vi "FormatWaveforms.vi"(0 "WaveformArray":sgl[](array[numeric]), 5 "logFileRef":refnum<k34>, 7 "log":bool, 9 "StreamHeader":T1, 11 "error in (no error)":errorcluster) -> (4 "Waveforms":sgl[][](array[numeric]), 6 "UpdateWaveforms":bool, 15 "error out":errorcluster)   [LabVIEW 2017]
uses:
  Controller/Support/StreamHeader.ctl
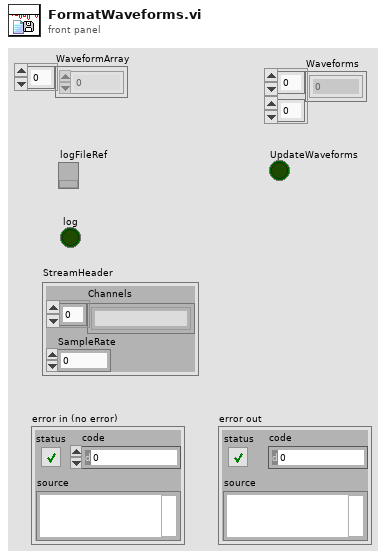
[diagram p1: front panel]
types:
  T1 = typedef "StreamHeader.ctl" = cluster{"Channels":string[], "SampleRate":i32}
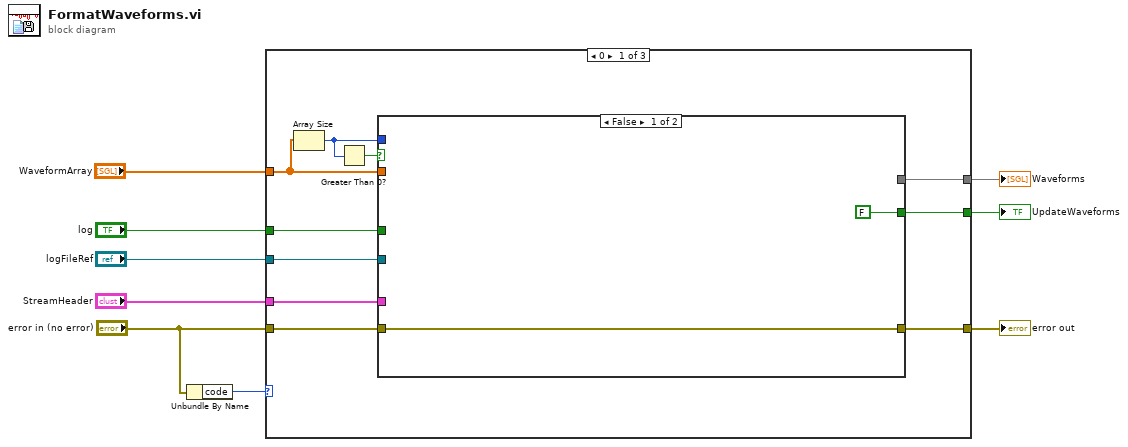
[diagram p0: block diagram]
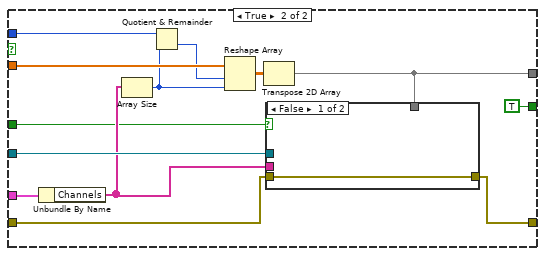
[diagram p2: hidden frame]
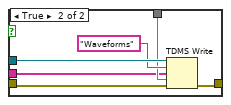
[diagram p3: hidden frame]
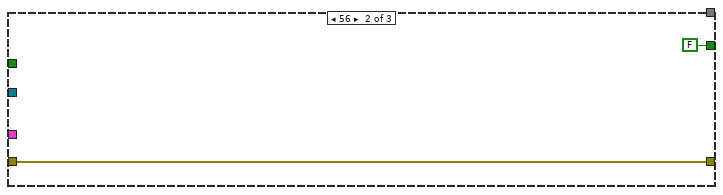
[diagram p4: hidden frame]
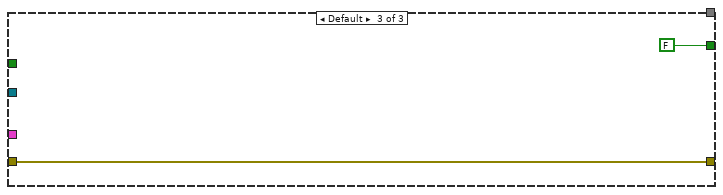
[diagram p5: hidden frame]
diagram:
  n1 = Unbundle By Name("error in (no error)") -> ("code"=w5:i32)
  n2 = case shown="0" w5 {
    tunnel: [w14 w43 w45] -> w3
    tunnel: "WaveformArray" -> [w19 _ _]
    tunnel: "StreamHeader" -> [w13 _ _]
    tunnel: "error in (no error)" -> [w15 w43 w45]
    tunnel: "logFileRef" -> [w16 _ _]
    tunnel: "log" -> [w12 _ _]
    tunnel: [w11 _ _] -> w1
    tunnel: [w10 FALSE FALSE] -> w2
    frame 0 {
      n3 = Array Size(array=w19) -> (size(s)=w18:i32)
      n4 = Greater Than 0?(x=w18) -> (x > 0?=w17:bool)
      n5 = case shown="False" w17 {
        tunnel: w19 -> [_ w34]
        tunnel: w18 -> [_ w31]
        tunnel: w13 -> [_ w28]
        tunnel: w16 -> [_ w30]
        tunnel: w15 -> [w21 w26]
        tunnel: [w21 w25] -> w14
        tunnel: w12 -> [_ w24]
        tunnel: [_ w23] -> w11
        tunnel: [FALSE TRUE] -> w10
        frame False {
        }
        frame True {
          n6 = Unbundle By Name(w28) -> ("Channels"=w27:string[])
          n7 = Array Size(array=w27) -> (size(s)=w29:i32)
          n8 = Quotient & Remainder(x=w31, y=w29) -> (floor(x/y)=w33:i32)  [unwired: 1 out]
          n9 = Reshape Array(w34, w33, w29) -> (w32:sgl[][])
          n10 = Transpose 2D Array(2D array=w32) -> (transposed array=w23:sgl[][])
          n11 = case shown="False" w24 {
            tunnel: w30 -> [_ w41]
            tunnel: w23 -> [_ w39]
            tunnel: w27 -> [_ w38]
            tunnel: w26 -> [w35 w37]
            tunnel: [w35 w36] -> w25
            frame False {
            }
            frame True {
              n12 = TDMS Write(0:w41, 5:"Waveforms" ("group name in (Untitled)"), 7:w38, 9:w39, 11:w37) -> (15:w36:errorcluster)  [unwired: 1 in, 3 out]
            }
          }
        }
      }
    }
    frame 56 {
    }
    frame Default {
    }
  }
  "error out" <- w3
  "UpdateWaveforms" <- w2
  "Waveforms" <- w1
